vi "Excel Set Cell Dimension.vi"(0 "report in":refnum<class "NI_report.lvclass">, 1 "width (-1)":dbl=-1.0 format="%0.2f", 2 "height (-1)":dbl=-1.0 format="%0.2f", 5 "measurement system":u16(ring) caption="measurement system (US)", 7 "start (-1, -1)":cluster{"row":i32, "column":i32}={"row"=-1, "column"=-1}, 9 "end (-1, -1)":cluster{"row":i32, "column":i32}={"row"=-1, "column"=-1}, 11 "error in (no error)":errorcluster, 12 "name (\"\")":string) -> (4 "report out":refnum<class "NI_report.lvclass">, 15 "error out":errorcluster)   [LabVIEW 2017, in "NI_Excel.lvclass"]
doc: "Sets the dimensions of the cells specified by the <B>start</B> and <B>end</B> clusters or by a named range."
uses:
  <vilib>/Utility/NIReport.llb/Excel/NI_Excel.lvclass
  <vilib>/Utility/NIReport.llb/NI_report.lvclass
  C:/Program Files (x86)/National Instruments/LabVIEW 2017/vi.lib/Utility/NIReport.llb/NI_report.lvclass
  <vilib>/Utility/NIReport.llb/Excel/NI_Excel.lvclass/NI_Excel.ctl
  <vilib>/addons/_office/NI_ReportGenerationToolkit.lvlib
  <vilib>/Utility/NIReport.llb/NI_ReportGenerationCore.lvlib
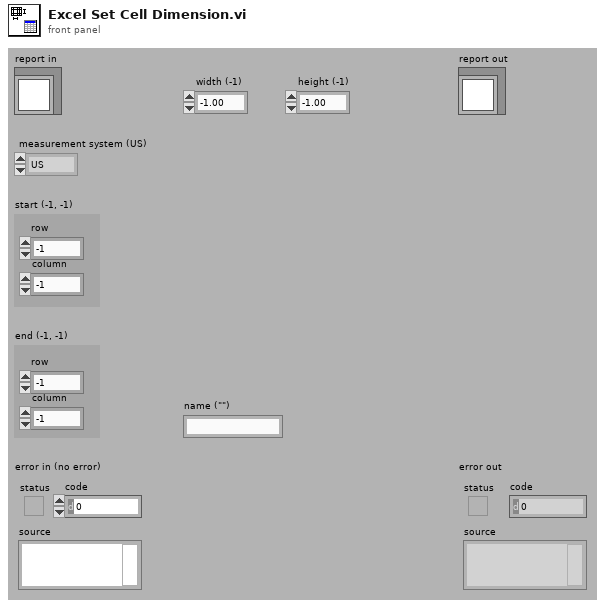
[diagram p1: front panel]
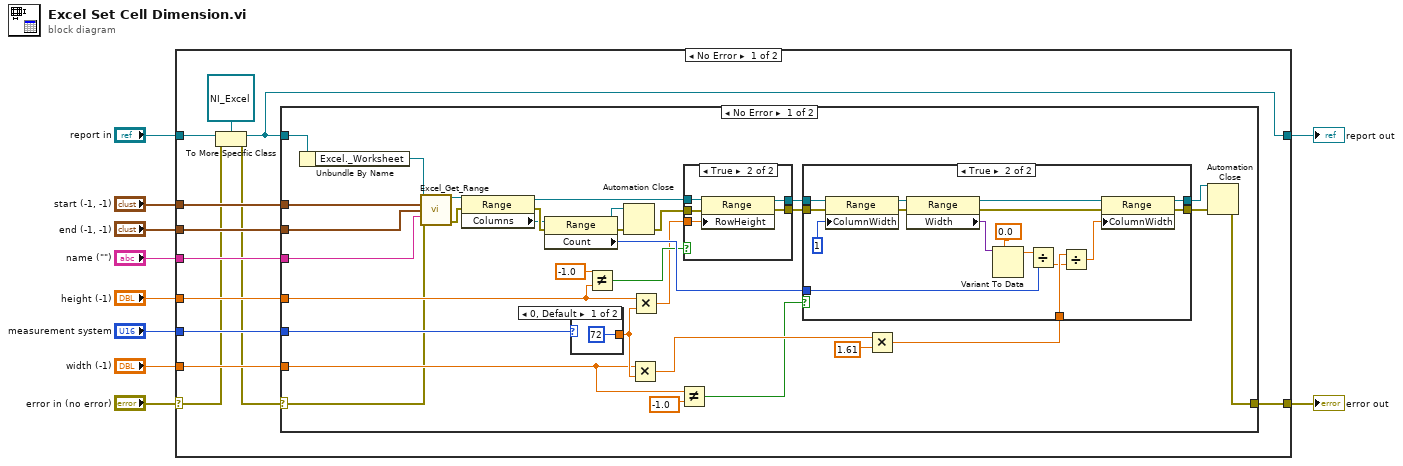
[diagram p0: block diagram]
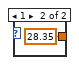
[diagram p4: hidden frame]
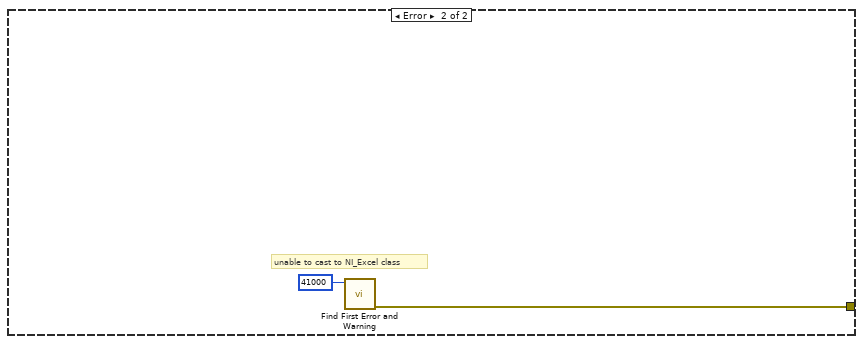
[diagram p5: hidden frame]
diagram:
  n1 = case shown="No Error" "error in (no error)" {
    selector: "error in (no error)" -> [w11 w85]
    tunnel: [w22 w85] -> w9
    tunnel: [w13 w84] -> w7
    tunnel: "report in" -> [w14 w84]
    tunnel: "start (-1, -1)" -> [w21 _]
    tunnel: "end (-1, -1)" -> [w20 _]
    tunnel: "name (\"\")" -> [w19 _]
    tunnel: "height (-1)" -> [w18 _]
    tunnel: "measurement system" -> [w17 _]
    tunnel: "width (-1)" -> [w16 _]
    frame No Error {
      n2 = To More Specific Class(target class=refnum<class "NI_Excel.lvclass"> refnum ("report in"), reference=w14, error in=w11) -> (specific class reference=w13:refnum<class "NI_Excel.lvclass">, error out=w12:errorcluster)
      n3 = case shown="No Error" w12 {
        selector: w12 -> [w23 _]
        tunnel: [w32 w82] -> w22
        tunnel: w21 -> [w31 _]
        tunnel: w20 -> [w30 _]
        tunnel: w19 -> [w29 _]
        tunnel: w18 -> [w28 _]
        tunnel: w17 -> [w27 _]
        tunnel: w16 -> [w26 _]
        tunnel: w13 -> [w24 _]
        frame No Error {
          n4 = Unbundle By Name(w24) -> ("Excel._Worksheet"=w25:refnum<k7>)
          n5 = call <vilib>:"Excel_Get_Range.vi"("Excel._Worksheet"=w25, "start"=w31, "end"=w30, "name"=w29, "error in (no error)"=w23) -> ("Range"=w34:refnum<k7>, "error out"=w35:errorcluster)  [unwired: 5 in, 4 out]
          n6 = property class="Range"(reference=w34, error in=w35) -> (reference out=w36:refnum<k7>, error out=w38:errorcluster, "Columns"=w37:refnum<k7>)
          n7 = property class="Range"(reference=w37, error in=w38) -> (reference out=w40:refnum<k7>, error out=w39:errorcluster, "Count"=w51:i32)
          n8 = case shown="0, Default" w27 {
            tunnel: [72 28.35] -> w48
            frame 0, Default {
            }
            frame 1 {
            }
          }
          n9 = Not Equal?(x=-1.0 ("y"), y=w28) -> (x != y?=w50:bool)
          n10 = Automation Close(3:w39, 5:w40) -> (0:w41:errorcluster)
          n11 = Multiply(x=w26, y=w48) -> (x*y=w52:dbl)
          n12 = Multiply(x=w28, y=w48) -> (x*y=w33:dbl)
          n13 = Not Equal?(x=w26, y=-1.0) -> (x != y?=w47:bool)
          n14 = case shown="True" w50 {
            tunnel: w33 -> [_ w61]
            tunnel: w36 -> [w56 w60]
            tunnel: w41 -> [w55 w59]
            tunnel: [w55 w58] -> w42
            tunnel: [w56 w57] -> w43
            frame False {
            }
            frame True {
              n15 = property class="Range"(reference=w60, error in=w59, "RowHeight"=w61) -> (reference out=w57:refnum<k7>, error out=w58:errorcluster)
            }
          }
          n16 = Multiply(x=w52, y=1.61) -> (x*y=w53:dbl)
          n17 = case shown="True" w47 {
            tunnel: w43 -> [w63 w79]
            tunnel: w42 -> [w62 w78]
            tunnel: [w62 w76] -> w44
            tunnel: [w63 w77] -> w45
            tunnel: w53 -> [_ w67]
            tunnel: w51 -> [_ w64]
            frame False {
            }
            frame True {
              n18 = property class="Range"(reference=w79, error in=w78, "ColumnWidth"=1) -> (reference out=w72:refnum<k7>, error out=w73:errorcluster)
              n19 = property class="Range"(reference=w72, error in=w73) -> (reference out=w70:refnum<k7>, error out=w71:errorcluster, "Width"=w69:variant)
              n20 = Variant To Data(type=0.0, Variant=w69) -> (data=w66:dbl)  [unwired: 1 in, 1 out]
              n21 = Divide(x=w66, y=w64) -> (x/y=w65:dbl)
              n22 = Divide(x=w67, y=w65) -> (x/y=w68:dbl)
              n23 = property class="Range"(reference=w70, error in=w71, "ColumnWidth"=w68) -> (reference out=w77:refnum<k7>, error out=w76:errorcluster)
            }
          }
          n24 = Automation Close(3:w44, 5:w45) -> (0:w32:errorcluster)
        }
        frame Error {
          # "unable to cast to NI_Excel class"
          n25 = call <vilib>:"Find First Error and Warning.vi"("error code"=41000) -> ("error out"=w82:errorcluster)  [unwired: 2 in, 4 out]
        }
      }
    }
    frame Error {
    }
  }
  "error out" <- w9
  "report out" <- w7
